vi "Get JKI CaseStructure Ref.vi"(8 "error in":errorcluster, 11 "VI Ref":refnum<vi>) -> (0 "error out":errorcluster, 2 "JKI Found":bool, 3 "CaseStructure Ref":refnum<vi>)   [LabVIEW 2020]
doc: "Looks for the presence of a Case Structure with a Terminal named \"Current State\" and assumes that the VI contains a JKI State Machine."
uses:
  <vilib>/Utility/traverseref.llb/TRef TravTarget.ctl
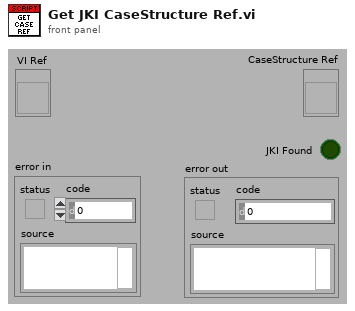
[diagram p1: front panel]
types:
  T1 = typedef "TRef TravTarget.ctl" = enum16{"FP", "BD", "Other"}
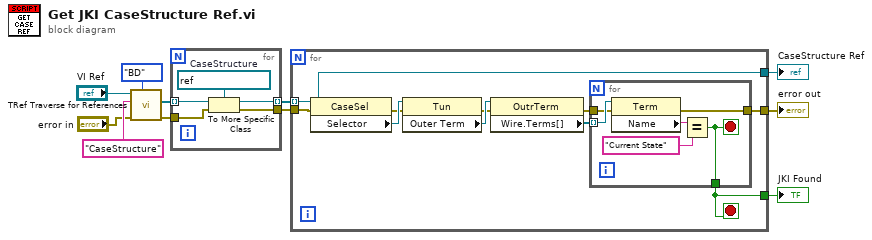
[diagram p0: block diagram]
diagram:
  n1 = call <vilib>:"TRef Traverse for References.vi"("Traverse Target"=TRef_TravTarget."BD", "error in (no error)"="error in", "Class Name"="CaseStructure", "VI Refnum"="VI Ref") -> ("error out"=w6:errorcluster, "References"=w9:refnum<vi>[])  [unwired: 1 in, 5 out]
  n2 = for {
    tunnel: w9 -> [w16] mode=indexing
    tunnel: [w14] -> w10 mode=indexing
    tunnel: w6 -> [w13]
    tunnel: [w12] -> w5
    w15 = refnum<vi> refnum  # CaseStructure
    n3 = To More Specific Class(target class=w15, reference=w16, error in=w13) -> (specific class reference=w14:refnum<vi>, error out=w12:errorcluster)
  }
  n4 = for {
    tunnel: w10 -> [w17] mode=indexing
    tunnel: [w17] -> w3
    tunnel: w5 -> [w20]
    tunnel: [w19] -> w2
    tunnel: [w18] -> w1
    stop <- w18 stop-if-true
    n5 = property class="CaseSel"(reference=w17, error in=w20) -> (error out=w25:errorcluster, "Selector"=w26:refnum<vi>)  [unwired: 1 out]
    n6 = property class="Tun"(reference=w26, error in=w25) -> (error out=w23:errorcluster, "Outer Term"=w24:refnum<vi>)  [unwired: 1 out]
    n7 = property class="OutrTerm"(reference=w24, error in=w23) -> (error out=w21:errorcluster, "Wire.Terms[]"=w22:refnum<vi>[])  [unwired: 1 out]
    n8 = for {
      tunnel: w22 -> [w32] mode=indexing
      tunnel: w21 -> [w31]
      tunnel: [w28] -> w18
      tunnel: [w27] -> w19
      stop <- w28 stop-if-true
      n9 = property class="Term"(reference=w32, error in=w31) -> (error out=w27:errorcluster, "Name"=w30:string)  [unwired: 1 out]
      n10 = Equal?(x=w30, y="Current State") -> (x = y?=w28:bool)
    }
  }
  "CaseStructure Ref" <- w3
  "error out" <- w2
  "JKI Found" <- w1
